vi "Start up.vi"() -> ()   [LabVIEW 2021]
uses:
  Libraries/User Interface/Hardware Selection Command.ctl
  Libraries/Database/Database.lvlib
  Libraries/CAN/CAN.lvlib
  Libraries/DAQ Hardware/DAQ Hardware.lvlib
  Libraries/DAQ IO/DAQ IO.lvlib
  Libraries/ARINC/ARINC.lvlib
  Libraries/DC PWS/DC PWS.lvlib
  Libraries/DMM/DMM.lvlib
  Libraries/Func Generator/Func Generator.lvlib
  Libraries/Oscilloscope/Oscilloscope.lvlib
  Libraries/S-Matrix/S-Matrix.lvlib
  Libraries/User Interface/User Interface.lvlib
  Libraries/Environment Chamber/Environment Chamber.lvlib
panel:
  out "error out":errorcluster
  in  "error in (no error)":errorcluster
  # "Start up"
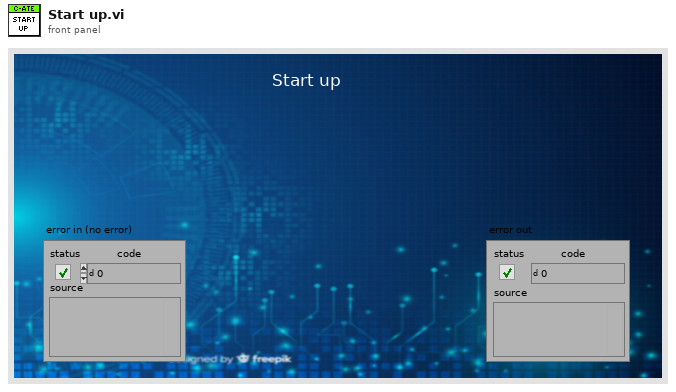
[diagram p1: front panel]
types:
  T1 = typedef "User Interface.lvlib/Hardware Selection Command.ctl" = enum16{"Init", "Read", "Write", "Close"}
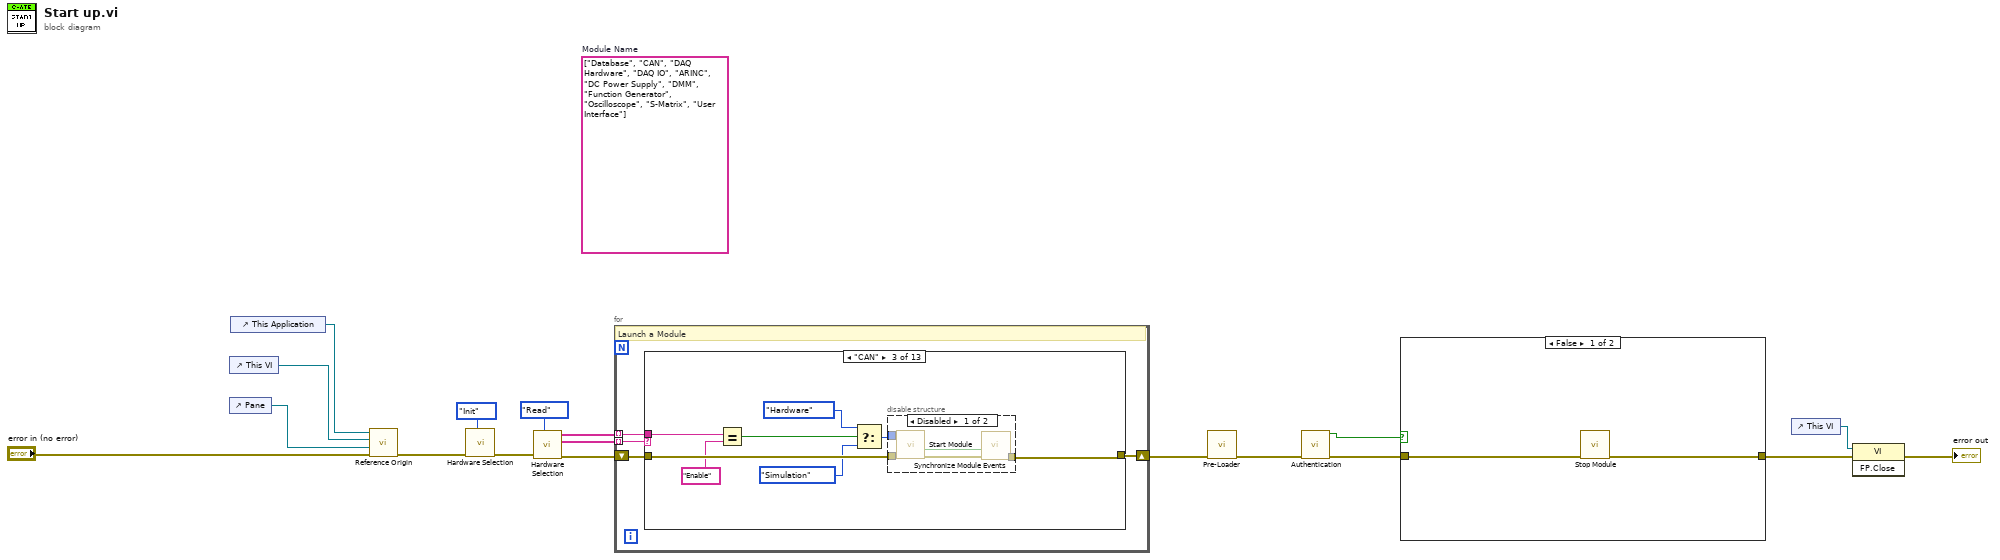
[diagram p0: block diagram]
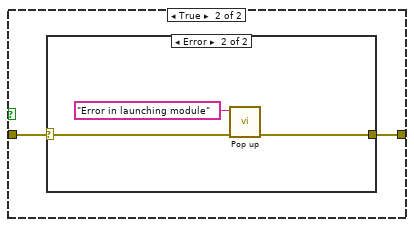
[diagram p2: hidden frame]
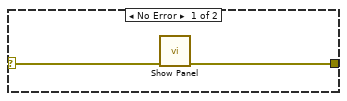
[diagram p3: hidden frame]
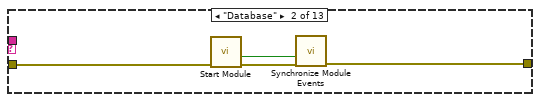
[diagram p5: hidden frame]
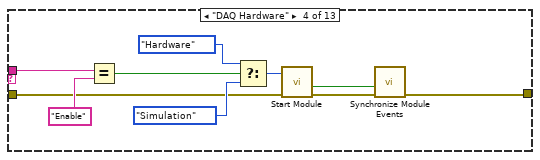
[diagram p7: hidden frame]
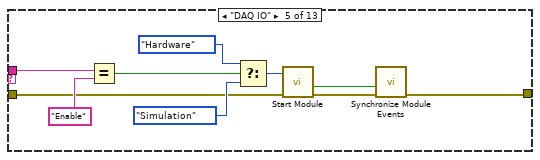
[diagram p8: hidden frame]
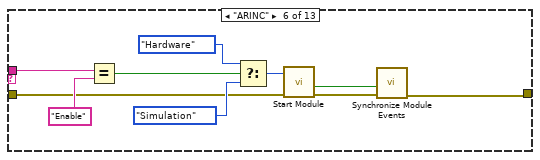
[diagram p9: hidden frame]
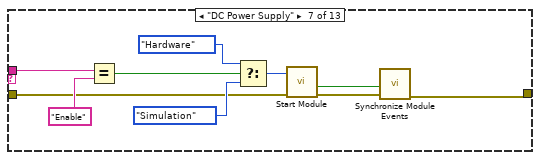
[diagram p10: hidden frame]
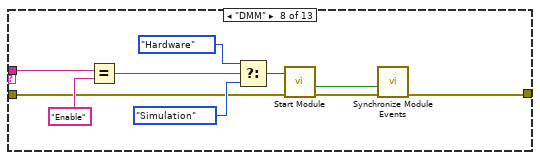
[diagram p11: hidden frame]
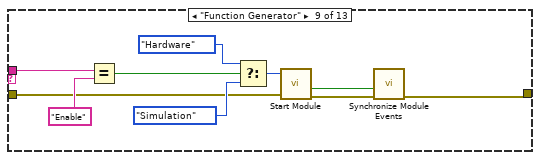
[diagram p12: hidden frame]
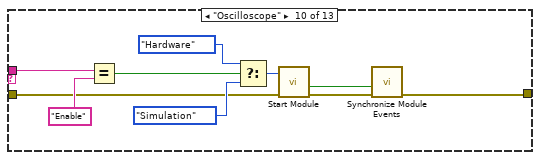
[diagram p13: hidden frame]
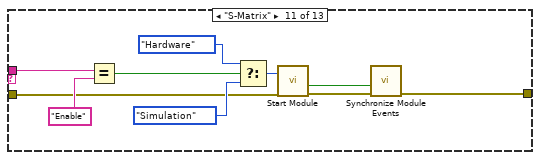
[diagram p14: hidden frame]
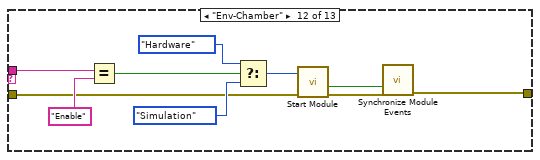
[diagram p15: hidden frame]
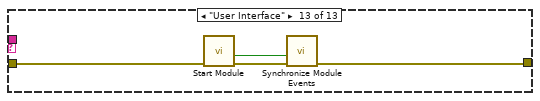
[diagram p16: hidden frame]
diagram:
  (unwired) string[] ["Database", "CAN", "DAQ Hardware", "DAQ IO", "ARINC", "DC Power Supply", "DMM", "Function Generator", "Oscilloscope", "S-Matrix", "User Interface"]  # Module Name
  n1 = control-ref of="This VI"() -> (w4:refnum<vi>)
  n2 = control-ref of="Pane"() -> (w16:refnum<vi>)
  n3 = control-ref of="This Application"() -> (w17:refnum<vi>)
  n4 = call "Reference Origin.vi"("error in (no error)"="error in (no error)", "Pane"=w16, "This VI"=w4, "This Application"=w17) -> ("error out"=w3:errorcluster)  [unwired: 6 in, 1 out]
  n5 = call "Hardware Selection.vi"("Command"=Hardware_Selection_Command."Init", "error in (no error)"=w3) -> ("error out"=w11:errorcluster)  [unwired: 7 in, 2 out]
  n6 = call "Hardware Selection.vi"("Command"=Hardware_Selection_Command."Read", "error in (no error)"=w11) -> ("error out"=w13:errorcluster, "Module Name"=w12:string[], "Hardware Selection"=w14:string[])  [unwired: 7 in]
  n7 = for {
    tunnel: w12 -> [w22] mode=indexing
    tunnel: w14 -> [w21] mode=indexing
    shift-right: [w19] -> w2
    shift-left: w13 -> [w20]
    # "Launch a Module"
    n8 = case shown="\"CAN\"" w22 {
      tunnel: w21 -> [_ _ w33 w50 w60 w70 w80 w90 w100 w110 w120 w130 _]
      tunnel: w20 -> [w23 w25 w35 w43 w53 w63 w73 w83 w92 w102 w112 w123 w132]
      tunnel: [w23 w24 w34 w42 w52 w61 w71 w82 w91 w101 w111 w122 w131] -> w19
      frame "False", Default {
      }
      frame "Database" {
        n9 = call "Start Module.vi"("error in"=w25) -> ("error out"=w26:errorcluster, "Wait for Event Sync?"=w27:bool)  [unwired: 7 in, 2 out]
        n10 = call "Synchronize Module Events.vi"("error in"=w26, "Wait for Event Sync?"=w27) -> ("error out"=w24:errorcluster)  [unwired: 9 in]
      }
      frame "CAN" {
        n11 = Equal?(x=w33, y="Enable") -> (x = y?=w31:bool)
        n12 = Select(t=enum16{"Hardware", "Simulation"}."Hardware" ("DAQ Type"), s=w31, f=enum16{"Hardware", "Simulation"}."Simulation" ("DAQ Type")) -> (s? t:f=w28:enum16{"Hardware", "Simulation"})
        n13 = disable-structure shown="Disabled" {
          disable-tunnel: w35 -> [w39 _]
          disable-tunnel: [w38 _] -> w34
          disable-tunnel: w28 -> [w36 _]
          frame Disabled {
            n14 = call "Start Module.vi"("error in"=w39, "DAQ Type"=w36) -> ("error out"=w37:errorcluster, "Wait for Event Sync?"=w40:bool)  [unwired: 6 in, 2 out]
            n15 = call "Synchronize Module Events.vi"("error in"=w37, "Wait for Event Sync?"=w40) -> ("error out"=w38:errorcluster)  [unwired: 9 in]
          }
          frame Enabled {
          }
        }
      }
      frame "DAQ Hardware" {
        n16 = Equal?(x=w50, y="Enable") -> (x = y?=w48:bool)
        n17 = Select(t=enum16{"Hardware", "Simulation"}."Hardware" ("DAQ Type"), s=w48, f=enum16{"Hardware", "Simulation"}."Simulation" ("DAQ Type")) -> (s? t:f=w41:enum16{"Hardware", "Simulation"})
        n18 = call "Start Module.vi"("error in"=w43, "DAQ Type"=w41) -> ("error out"=w44:errorcluster, "Wait for Event Sync?"=w45:bool)  [unwired: 6 in, 2 out]
        n19 = call "Synchronize Module Events.vi"("error in"=w44, "Wait for Event Sync?"=w45) -> ("error out"=w42:errorcluster)  [unwired: 9 in]
      }
      frame "DAQ IO" {
        n20 = Equal?(x=w60, y="Enable") -> (x = y?=w58:bool)
        n21 = Select(t=enum16{"Hardware", "Simulation"}."Hardware" ("DAQ Type"), s=w58, f=enum16{"Hardware", "Simulation"}."Simulation" ("DAQ Type")) -> (s? t:f=w51:enum16{"Hardware", "Simulation"})
        n22 = call "Start Module.vi"("error in"=w53, "DAQ Type"=w51) -> ("error out"=w54:errorcluster, "Wait for Event Sync?"=w55:bool)  [unwired: 6 in, 2 out]
        n23 = call "Synchronize Module Events.vi"("error in"=w54, "Wait for Event Sync?"=w55) -> ("error out"=w52:errorcluster)  [unwired: 9 in]
      }
      frame "ARINC" {
        n24 = Equal?(x=w70, y="Enable") -> (x = y?=w68:bool)
        n25 = Select(t=enum16{"Hardware", "Simulation"}."Hardware" ("DAQ Type"), s=w68, f=enum16{"Hardware", "Simulation"}."Simulation" ("DAQ Type")) -> (s? t:f=w62:enum16{"Hardware", "Simulation"})
        n26 = call "Start Module.vi"("error in"=w63, "DAQ Type"=w62) -> ("error out"=w64:errorcluster, "Wait for Event Sync?"=w65:bool)  [unwired: 6 in, 2 out]
        n27 = call "Synchronize Module Events.vi"("error in"=w64, "Wait for Event Sync?"=w65) -> ("error out"=w61:errorcluster)  [unwired: 9 in]
      }
      frame "DC Power Supply" {
        n28 = Equal?(x=w80, y="Enable") -> (x = y?=w78:bool)
        n29 = Select(t=enum16{"Hardware", "Simulation"}."Hardware" ("DAQ Type"), s=w78, f=enum16{"Hardware", "Simulation"}."Simulation" ("DAQ Type")) -> (s? t:f=w72:enum16{"Hardware", "Simulation"})
        n30 = call "Start Module.vi"("error in"=w73, "DAQ Type"=w72) -> ("error out"=w74:errorcluster, "Wait for Event Sync?"=w75:bool)  [unwired: 6 in, 2 out]
        n31 = call "Synchronize Module Events.vi"("error in"=w74, "Wait for Event Sync?"=w75) -> ("error out"=w71:errorcluster)  [unwired: 9 in]
      }
      frame "DMM" {
        n32 = Equal?(x=w90, y="Enable") -> (x = y?=w88:bool)
        n33 = Select(t=enum16{"Hardware", "Simulation"}."Hardware" ("DAQ Type"), s=w88, f=enum16{"Hardware", "Simulation"}."Simulation" ("DAQ Type")) -> (s? t:f=w81:enum16{"Hardware", "Simulation"})
        n34 = call "Start Module.vi"("error in"=w83, "DAQ Type"=w81) -> ("error out"=w84:errorcluster, "Wait for Event Sync?"=w85:bool)  [unwired: 6 in, 2 out]
        n35 = call "Synchronize Module Events.vi"("error in"=w84, "Wait for Event Sync?"=w85) -> ("error out"=w82:errorcluster)  [unwired: 9 in]
      }
      frame "Function Generator" {
        n36 = Equal?(x=w100, y="Enable") -> (x = y?=w98:bool)
        n37 = Select(t=enum16{"Hardware", "Simulation"}."Hardware" ("DAQ Type"), s=w98, f=enum16{"Hardware", "Simulation"}."Simulation" ("DAQ Type")) -> (s? t:f=w93:enum16{"Hardware", "Simulation"})
        n38 = call "Start Module.vi"("error in"=w92, "DAQ Type"=w93) -> ("error out"=w94:errorcluster, "Wait for Event Sync?"=w95:bool)  [unwired: 6 in, 2 out]
        n39 = call "Synchronize Module Events.vi"("error in"=w94, "Wait for Event Sync?"=w95) -> ("error out"=w91:errorcluster)  [unwired: 9 in]
      }
      frame "Oscilloscope" {
        n40 = Equal?(x=w110, y="Enable") -> (x = y?=w108:bool)
        n41 = Select(t=enum16{"Hardware", "Simulation"}."Hardware" ("DAQ Type"), s=w108, f=enum16{"Hardware", "Simulation"}."Simulation" ("DAQ Type")) -> (s? t:f=w103:enum16{"Hardware", "Simulation"})
        n42 = call "Start Module.vi"("error in"=w102, "DAQ Type"=w103) -> ("error out"=w104:errorcluster, "Wait for Event Sync?"=w105:bool)  [unwired: 6 in, 2 out]
        n43 = call "Synchronize Module Events.vi"("error in"=w104, "Wait for Event Sync?"=w105) -> ("error out"=w101:errorcluster)  [unwired: 9 in]
      }
      frame "S-Matrix" {
        n44 = Equal?(x=w120, y="Enable") -> (x = y?=w118:bool)
        n45 = Select(t=enum16{"Hardware", "Simulation"}."Hardware" ("DAQ Type"), s=w118, f=enum16{"Hardware", "Simulation"}."Simulation" ("DAQ Type")) -> (s? t:f=w113:enum16{"Hardware", "Simulation"})
        n46 = call "Start Module.vi"("error in"=w112, "DAQ Type"=w113) -> ("error out"=w114:errorcluster, "Wait for Event Sync?"=w115:bool)  [unwired: 6 in, 2 out]
        n47 = call "Synchronize Module Events.vi"("error in"=w114, "Wait for Event Sync?"=w115) -> ("error out"=w111:errorcluster)  [unwired: 9 in]
      }
      frame "Env-Chamber" {
        n48 = Equal?(x=w130, y="Enable") -> (x = y?=w128:bool)
        n49 = Select(t=enum16{"Hardware", "Simulation"}."Hardware" ("DAQ Type"), s=w128, f=enum16{"Hardware", "Simulation"}."Simulation" ("DAQ Type")) -> (s? t:f=w121:enum16{"Hardware", "Simulation"})
        n50 = call "Start Module.vi"("error in"=w123, "DAQ Type"=w121) -> ("error out"=w124:errorcluster, "Wait for Event Sync?"=w125:bool)  [unwired: 6 in, 2 out]
        n51 = call "Synchronize Module Events.vi"("error in"=w124, "Wait for Event Sync?"=w125) -> ("error out"=w122:errorcluster)  [unwired: 9 in]
      }
      frame "User Interface" {
        n52 = call "Start Module.vi"("error in"=w132) -> ("error out"=w133:errorcluster, "Wait for Event Sync?"=w134:bool)  [unwired: 7 in, 2 out]
        n53 = call "Synchronize Module Events.vi"("error in"=w133, "Wait for Event Sync?"=w134) -> ("error out"=w131:errorcluster)  [unwired: 9 in]
      }
    }
  }
  n54 = call "Pre-Loader.vi"("error in (no error)"=w2) -> ("error out"=w1:errorcluster)  [unwired: 10 in]
  n55 = call "Authentication.vi"("error in (no error)"=w1) -> ("error out"=w6:errorcluster, "Match?"=w5:bool)  [unwired: 9 in]
  n56 = case shown="False" w5 {
    tunnel: [w135 w138] -> w9
    tunnel: w6 -> [w136 w137]
    frame False {
      n57 = call "Stop Module.vi"("error in"=w136) -> ("error out"=w135:errorcluster)  [unwired: 10 in]
    }
    frame True {
      n58 = case shown="Error" w137 {
        selector: w137 -> [w140 w143]
        tunnel: [w139 w142] -> w138
        frame No Error {
          n59 = call "Show Panel.vi"("error in (no error)"=w140) -> ("error out"=w139:errorcluster)  [unwired: 10 in]
        }
        frame Error {
          n60 = call "Pop up.vi"("error in (no error)"=w143, "Message In"="Error in launching module") -> ("error out"=w142:errorcluster)  [unwired: 7 in, 2 out]
        }
      }
    }
  }
  n61 = control-ref of="This VI"() -> (w7:refnum<vi>)
  n62 = invoke class="VI" method="FP.Close"(reference=w7, error in=w9) -> (error out=→"error out":errorcluster)  [unwired: 1 in, 2 out]
